vi "UsrProfiles-Obtain users.vi"(8 "error in":errorcluster) -> (0 "error out":errorcluster, 2 "User names":string[](array[string]))   [LabVIEW 2020]
uses:
  Typedefs/Which path.ctl
  <userlib>/_OpenG.lib/array/array.llb/Remove Duplicates from 1D Array (String)__ogtk.vi
  <userlib>/_OpenG.lib/array/array.llb/Sort 1D Array (String)__ogtk.vi
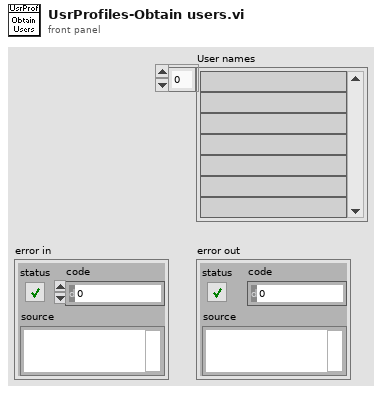
[diagram p1: front panel]
types:
  T1 = typedef "Which path.ctl" = enum16{"Configuration Files", "Calibration Files", "Images", "Setup.ini", "Loaded User profile.ini", "User's-Previous session.ini", "New user profile.ini", "Selected User profile.ini", "User profiles folder", "Power meter scaling.txt", "FOV Cal.ini", "Calibration.ini"}
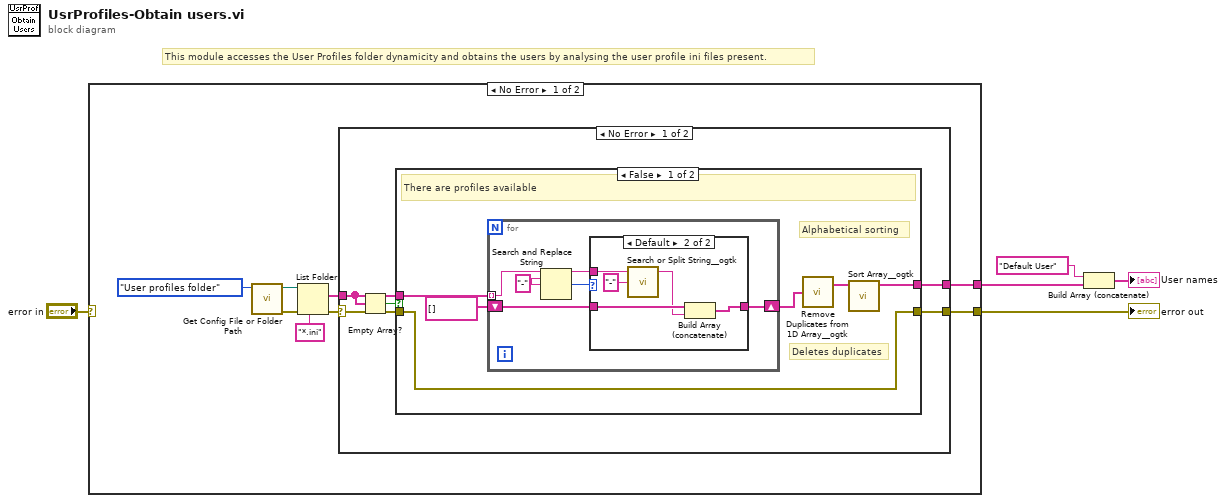
[diagram p0: block diagram]
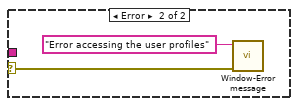
[diagram p4: hidden frame]
diagram:
  # "This module accesses the User Profiles folder dynamicity and obtains the users by analysing the user profile ini files present."
  n1 = case shown="No Error" "error in" {
    selector: "error in" -> [_ w40]
    tunnel: [w8 w40] -> w5
    tunnel: [w7 _] -> w2
    frame No Error {
      n2 = call "Get Config File or Folder Path.vi"("Which file or folder?"=Which_path."User profiles folder") -> ("Error Out"=w11:errorcluster, "File Path"=w12:path)  [unwired: 8 in, 1 out]
      n3 = List Folder(path=w12, pattern="*.ini", error in=w11) -> (filenames=w9:string[], error out=w10:errorcluster)  [unwired: 1 in, 2 out]
      n4 = case shown="No Error" w10 {
        selector: w10 -> [w17 w39]
        tunnel: w9 -> [w15 _]
        tunnel: [w16 _] -> w8
        tunnel: [w14 _] -> w7
        frame No Error {
          n5 = Empty Array?(array=w15) -> (empty?=w18:bool)
          n6 = case shown="False" w18 {
            tunnel: w15 -> [w24 _]
            tunnel: w17 -> [w23 w37]
            tunnel: [w23 w37] -> w16
            tunnel: [w19 _] -> w14
            frame False {
              # "Deletes duplicates"
              # "Alphabetical sorting"
              # "There are profiles available"
              n7 = for {
                tunnel: w24 -> [w27] mode=indexing
                shift-right: [w29] -> w21
                shift-left: string[] [] -> [w30]
                w28 = "-" ("search string/char (-)")
                n8 = Search and Replace String(input string=w27, search string=w28, replace string=w28) -> (result string=w26:string, number of replacements=w25:i32)  [unwired: 5 in, 2 out]
                n9 = case shown="Default" w25 {
                  tunnel: w30 -> [w31 w35]
                  tunnel: [w31 w34] -> w29
                  tunnel: w26 -> [_ w33]
                  frame 0 {
                  }
                  frame Default {
                    n10 = call <userlib>:"Search or Split String__ogtk.vi"("search string/char (-)"="-", "string"=w33) -> ("substring before match"=w32:string)  [unwired: 1 in, 2 out]
                    n11 = Build Array (concatenate)(w35, w32) -> (w34:string[])
                  }
                }
              }
              n12 = call-poly <userlib>:"Remove Duplicates from 1D Array__ogtk.vi"("Input Array"=w21) -> ("Output Array"=w20:string[])  [unwired: 1 out]
              n13 = call-poly <userlib>:"Sort Array__ogtk.vi"("Array in"=w20) -> ("Sorted Array out"=w19:string[])  [unwired: 9 in, 1 out]
            }
            frame True {
              # "No profiles available. Even the default profile is missing."
            }
          }
        }
        frame Error {
          n14 = call "Window-Error message.vi"("error in (no error)"=w39, "Message"="Error accessing the user profiles") -> ()  [unwired: 9 in, 1 out]
        }
      }
    }
    frame Error {
    }
  }
  "error out" <- w5
  n15 = Build Array (concatenate)("Default User", w2) -> (→"User names":string[])
